vi "Get Net Phi.vi"(8 "error in":errorcluster, 11 "Orient3d":refnum<class "Orient3d Class.lvclass">) -> (0 "error out":errorcluster, 2 "phi":dbl)   [LabVIEW 2011]
uses:
  Orient3d Class/Orient3d Class.lvclass
  Vec3d Class/Vec3d Class.lvclass
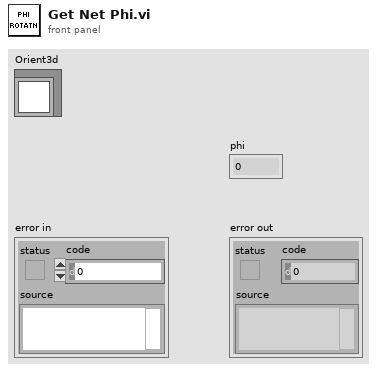
[diagram p1: front panel]
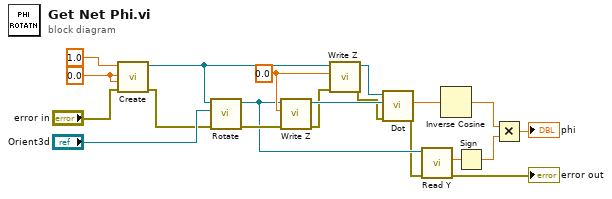
[diagram p0: block diagram]
diagram:
  w10 = 0.0 ("Z")
  w19 = 0.0 ("Y")
  n1 = call "Create.vi"("error in"="error in", "Z"=w19, "Y"=w19, "X"=1.0) -> ("error out"=w16:errorcluster, "Vec3d Class out"=w14:refnum<class "Vec3d Class.lvclass">)  [unwired: 6 in]
  n2 = call-dynamic "Rotate.vi"("error in"=w16, "Orient3d in"="Orient3d", "Vec3d in"=w14) -> ("error out"=w12:errorcluster, "Vec3d out"=w9:refnum<class "Vec3d Class.lvclass">)  [unwired: 7 in]
  n3 = call-dynamic "Write Z.vi"("error in (no error)"=w12, "Z"=w10, "Vec3d Class in"=w9) -> ("error out"=w3:errorcluster, "Vec3d Class out"=w11:refnum<class "Vec3d Class.lvclass">)  [unwired: 7 in]
  n4 = call-dynamic "Write Z.vi"("error in (no error)"=w3, "Z"=w10, "Vec3d Class in"=w14) -> ("error out"=w2:errorcluster, "Vec3d Class out"=w13:refnum<class "Vec3d Class.lvclass">)  [unwired: 7 in]
  n5 = call "Dot.vi"("error in"=w2, "Vec3d in 2"=w11, "Vec3d in 1"=w13) -> ("error out"=w4:errorcluster, "Dot Product"=w15:dbl)  [unwired: 7 in]
  n6 = call-dynamic "Read Y.vi"("error in (no error)"=w4, "Vec3d Class in"=w9) -> ("error out"=→"error out":errorcluster, "Y"=w8:dbl)  [unwired: 7 in, 1 out]
  n7 = Inverse Cosine(1:w15) -> (0:w6:dbl)
  n8 = Sign(1:w8) -> (0:w7:dbl)
  n9 = Multiply(x=w6, y=w7) -> (x*y=→"phi":dbl)
